vi "Get Voltage and SoC.vi"(0 "reference in":refnum<class "Battery.lvclass">, 5 "Error In":errorcluster) -> (14 "reference out":refnum<class "Battery.lvclass">, 16 "Cell Voltage (V)":dbl, 19 "Error Out":errorcluster)   [LabVIEW 2023, in "Battery.lvclass"]
uses:
  Battery.lvclass
panel:
  out "SoC (%)":dbl
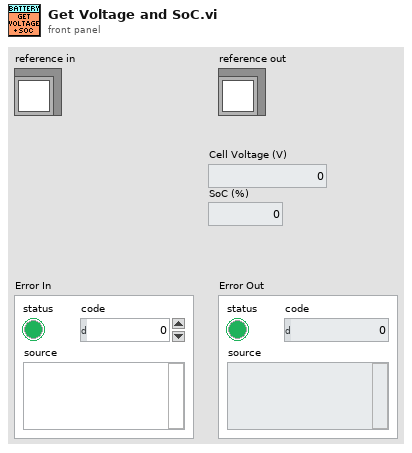
[diagram p1: front panel]
types:
  T1 = typedef "Battery.lvclass/ObjectAttributes.ctl" = cluster{"Mode":enum16{"Disconnected", "Charging", "Discharging"}, "Discharge Switch":bool, "Allow Charging":bool, "Cell Voltage (V)":dbl, "Cell Current (A)":dbl, "SoC (%)":dbl, "Nominal Voltage (V)":dbl, "Model Index":i32, "Charge Model":cluster{"Voltage (V)":dbl[], "Current (A)":dbl[], "SoC (%)":dbl[]}, "Discharge Model":cluster{"Voltage (V)":dbl[], "Current (A)":dbl[], "SoC (%)":dbl[]}, "Simulation Error":errorcluster}
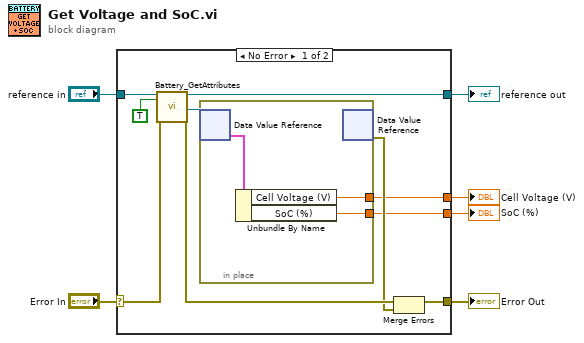
[diagram p0: block diagram]
diagram:
  n1 = case shown="No Error" "Error In" {
    selector: "Error In" -> [w16 w21]
    tunnel: [w14 w21] -> w5
    tunnel: [w11 w20] -> w3
    tunnel: "reference in" -> [w12 w20]
    tunnel: [w8 _] -> w2
    tunnel: [w7 _] -> w1
    frame No Error {
      n2 = call "Battery_GetAttributes.vi"("reference in"=w12, "OnlyGetDvrReference(False)"=TRUE, "Error In"=w16) -> ("reference out"=w11:refnum<class "Battery.lvclass">, "DataRef"=w10:refnum<data-value>, "Error Out"=w15:errorcluster)  [unwired: 13 in, 1 out]
      n3 = in-place {
        in-place-border: [w19] -> w8
        in-place-border: [w17] -> w7
        n4 = in-place-dvr #1(w10) -> (w18:T1)  [unwired: 1 out]
        n5 = Unbundle By Name(w18) -> ("Cell Voltage (V)"=w19:dbl, "SoC (%)"=w17:dbl)
        n6 = in-place-dvr #1() -> (w13:errorcluster)  [unwired: 1 in, 1 out]
      }
      n7 = Merge Errors(w15, w13) -> (w14:errorcluster)
    }
    frame Error {
    }
  }
  "Error Out" <- w5
  "reference out" <- w3
  "Cell Voltage (V)" <- w2
  "SoC (%)" <- w1
